vi "MSEncoder SubVI WfmCodeAccess PhaseScan.vi"(8 "error in":errorcluster, 9 "Data in":T1, 11 "MSEncoder in":refnum<class "MSEncoder.lvclass">) -> (0 "error out":errorcluster, 3 "MSEncoder out":refnum<class "MSEncoder.lvclass">)   [LabVIEW 2018, in "MSEncoder.lvclass"]
uses:
  MSEncoder.lvclass
  MSEncoder.lvclass/MSEncoder.ctl
  WfmDataAccessor/WfmDataAccessor.lvclass
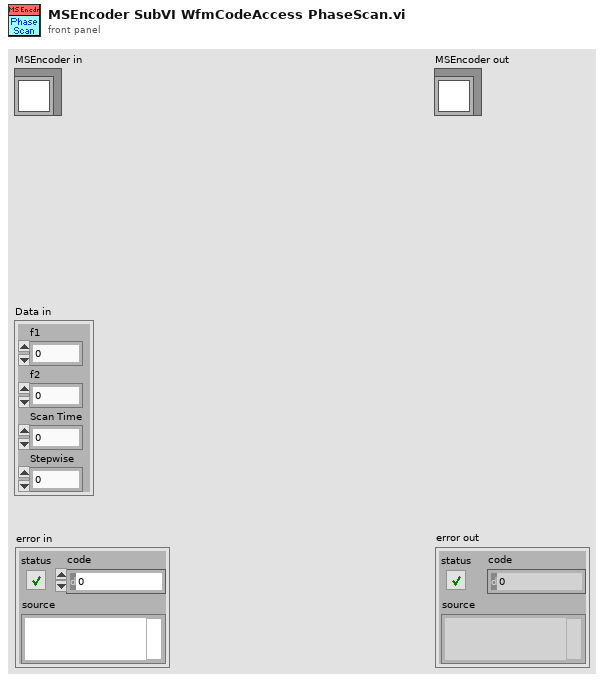
[diagram p1: front panel]
types:
  T1 = cluster{"f1":ext, "f2":ext, "Scan Time":ext, "Stepwise":u32}
  T2 = cluster{"Data in":cluster{"f1":ext, "f2":ext, "Scan Time":ext, "Stepwise":u32}, "CycDiff":u64[], "Ratio":u16[], "1/Decyc":u32, "Decyc":u32}
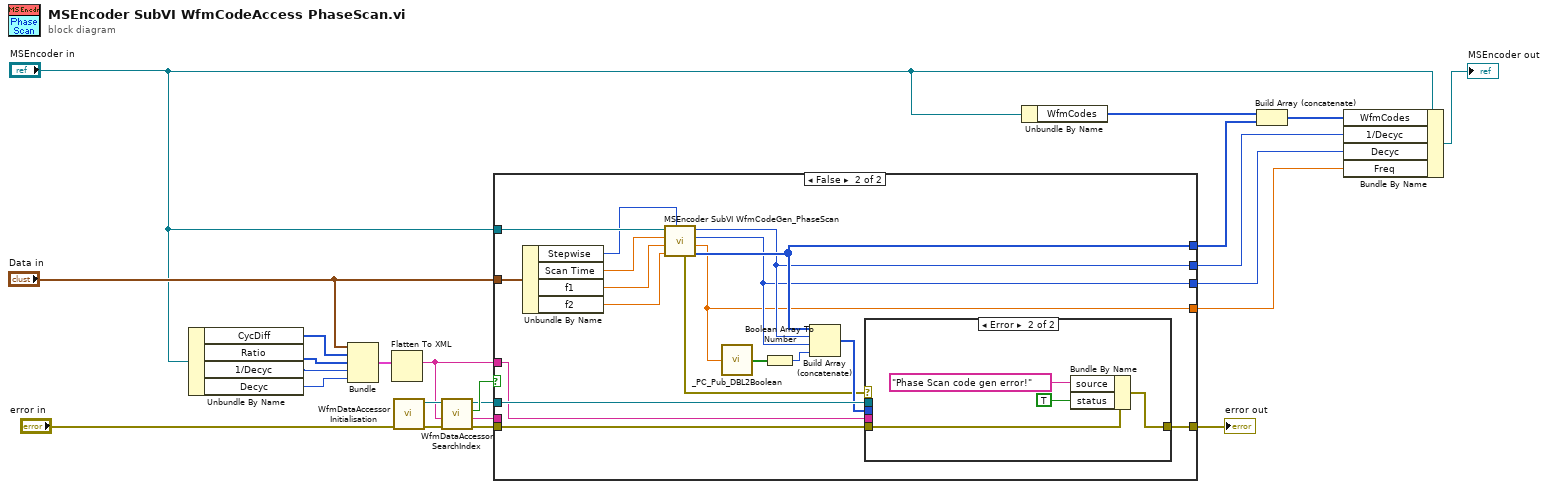
[diagram p0: block diagram]
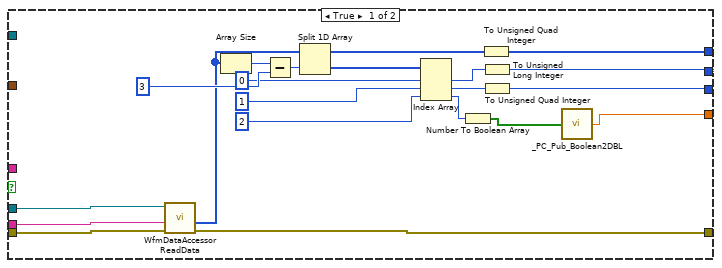
[diagram p2: hidden frame]
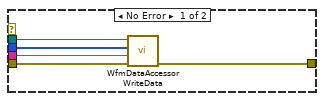
[diagram p3: hidden frame]
diagram:
  n1 = Unbundle By Name("MSEncoder in") -> ("CycDiff"=w18:u64[], "Ratio"=w19:u16[], "1/Decyc"=w20:u32, "Decyc"=w21:u32)
  n2 = Bundle("Data in"="Data in", "CycDiff"=w18, "Ratio"=w19, "1/Decyc"=w20, "Decyc"=w21) -> (w17:T2)  [unwired: 1 in]
  n3 = Flatten To XML(anything=w17) -> (xml string=w10:string)
  n4 = call "WfmDataAccessor Initialisation.vi"("error in (no error)"="error in") -> ("error out"=w11:errorcluster, "WfmDataAccessor out"=w12:refnum<class "WfmDataAccessor.lvclass">)  [unwired: 9 in]
  n5 = call-dynamic "WfmDataAccessor SearchIndex.vi"("error in (no error)"=w11, "XML in"=w10, "WfmDataAccessor in"=w12) -> ("error out"=w7:errorcluster, "filename"=w6:string, "Found"=w9:bool, "WfmDataAccessor out"=w8:refnum<class "WfmDataAccessor.lvclass">)  [unwired: 5 in]
  n6 = case shown="False" w9 {
    tunnel: "MSEncoder in" -> [_ w50]
    tunnel: "Data in" -> [_ w51]
    tunnel: [w25 w58] -> w13
    tunnel: [w38 w62] -> w16
    tunnel: [w32 w61] -> w15
    tunnel: [w34 w60] -> w14
    tunnel: [w24 w52] -> w1
    tunnel: w10 -> [_ w53]
    tunnel: w8 -> [w31 w59]
    tunnel: w7 -> [w30 w54]
    tunnel: w6 -> [w29 _]
    frame True {
      n7 = call-dynamic "WfmDataAccessor ReadData.vi"("error in (no error)"=w30, "Filename"=w29, "WfmDataAccessor in"=w31) -> ("error out"=w24:errorcluster, "WfmData"=w28:u64[])  [unwired: 6 in, 1 out]
      n8 = Array Size(array=w28) -> (size(s)=w44:i32)
      n9 = Subtract(x=w44, y=3) -> (x-y=w42:i32)
      n10 = Split 1D Array(array=w28, index=w42) -> (first subarray=w39:u64[], second subarray=w41:u64[])
      n11 = Index Array(array=w41, index #1=0 ("index"), index #2=1 ("index"), index #3=2 ("index")) -> (element #1=w33:u64, element #2=w35:u64, element #3=w27:u64)
      n12 = Number To Boolean Array(number=w27) -> (Boolean array=w26:bool[])
      n13 = To Unsigned Quad Integer(1:w39) -> (0:w38:u64[])
      n14 = To Unsigned Long Integer(number=w33) -> (unsigned 32bit integer=w32:u32)
      n15 = To Unsigned Quad Integer(1:w35) -> (0:w34:u64)
      n16 = call "_PC_Pub_Boolean2DBL.vi"("Boolean array"=w26) -> ("DBL"=w25:dbl)
    }
    frame False {
      n17 = Unbundle By Name(w51) -> ("Stepwise"=w49:u32, "Scan Time"=w48:ext, "f1"=w47:ext, "f2"=w46:ext)
      n18 = call "MSEncoder SubVI WfmCodeGen_PhaseScan.vi"("Stepwise"=w49, "f2"=w46, "f1"=w47, "Scan time"=w48, "MSEncoder.lvclass"=w50) -> ("WfmCode"=w62:u64[], "Actual Freq"=w58:dbl, "Decyc"=w60:u64, "1/Decyc"=w61:u32, "error out"=w45:errorcluster)  [unwired: 2 in]
      n19 = call "_PC_Pub_DBL2Boolean.vi"("DBL"=w58) -> ("Boolean array"=w57:bool[])
      n20 = Boolean Array To Number(Boolean array=w57) -> (number=w56:u64)
      n21 = Build Array (concatenate)(w62, w61, w60, w56) -> (w55:u64[])
      n22 = case shown="Error" w45 {
        tunnel: w59 -> [w67 _]
        tunnel: w55 -> [w66 _]
        tunnel: w54 -> [w65 w69]
        tunnel: w53 -> [w64 _]
        tunnel: [w63 w68] -> w52
        frame No Error {
          n23 = call-dynamic "WfmDataAccessor WriteData.vi"("error in (no error)"=w65, "XML"=w64, "WfmData"=w66, "WfmDataAccessor in"=w67) -> ("error out"=w63:errorcluster)  [unwired: 6 in, 1 out]
        }
        frame Error {
          n24 = Bundle By Name(cluster=w69, "source"="Phase Scan code gen error!", "status"=TRUE) -> (w68:errorcluster)
        }
      }
    }
  }
  "error out" <- w1
  n25 = Unbundle By Name("MSEncoder in") -> ("WfmCodes"=w23:u64[])
  n26 = Build Array (concatenate)(w23, w16) -> (w22:u64[])
  n27 = Bundle By Name(cluster="MSEncoder in", "WfmCodes"=w22, "1/Decyc"=w15, "Decyc"=w14, "Freq"=w13) -> (→"MSEncoder out":refnum<class "MSEncoder.lvclass">)
